vi "testNoError.vi"() -> ()   [LabVIEW 2019, in "AssertionTest.lvlib" / "AssertNoError.lvlib"]
uses:
  AssertNoError.lvlib
  Assertion/Assertion.lvlib
  Error/Error.lvlib
panel:
  out "error out":errorcluster
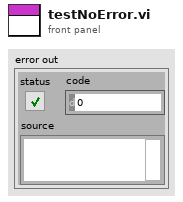
[diagram p1: front panel]
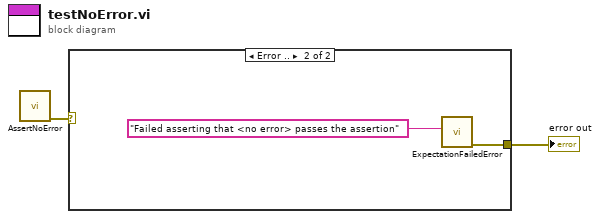
[diagram p0: block diagram]
diagram:
  n1 = call "AssertNoError.vi"() -> ("error out"=w2:errorcluster)  [unwired: 11 in]
  n2 = case shown="Error .." w2 {
    tunnel: [_ w3] -> w1
    frame No Error {
    }
    frame Error {
      n3 = call "ExpectationFailedError.vi"("Message"="Failed asserting that <no error> passes the assertion" ("error message (\"\")")) -> ("error out"=w3:errorcluster)  [unwired: 10 in]
    }
  }
  "error out" <- w1
